vi "rethinkdb_handshake3.vi"(6 "timeout ms (10000)":i32=10000, 8 "error in (no error)":errorcluster, 10 "auth client final":string="r=rOprNGfwEbeRWgbNEkqO%hvYDpWUa2RaTCAfuxFIlj)hNlF$k0,s=W22ZaJ0SNY7soEsUEjb6gQ==,i=4096", 11 "rethinkdb in":refnum<k5>) -> (0 "error out":errorcluster, 2 "auth server final":string, 3 "rethinkdb out":refnum<k5>)   [LabVIEW 2017]
uses:
  b9d4f6d7-50ba-4a66-8241-62e1aea0d02a.vi
  17f0a6fe-6775-4334-81ae-21231bb255b8.vi
  json/rethinkdb_json_from_cluster.vi
  json/rethinkdb_json_to_cluster.vi
  json/rethinkdb_json_type_cast.vi
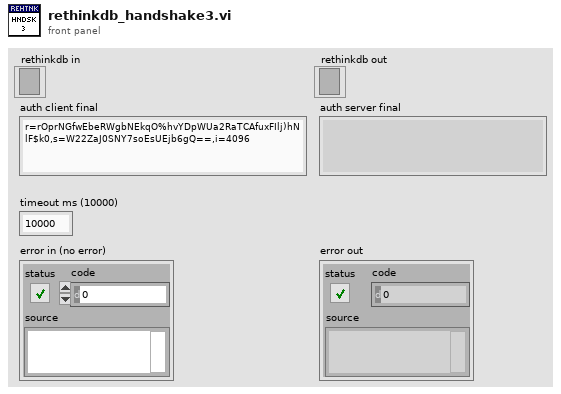
[diagram p1: front panel]
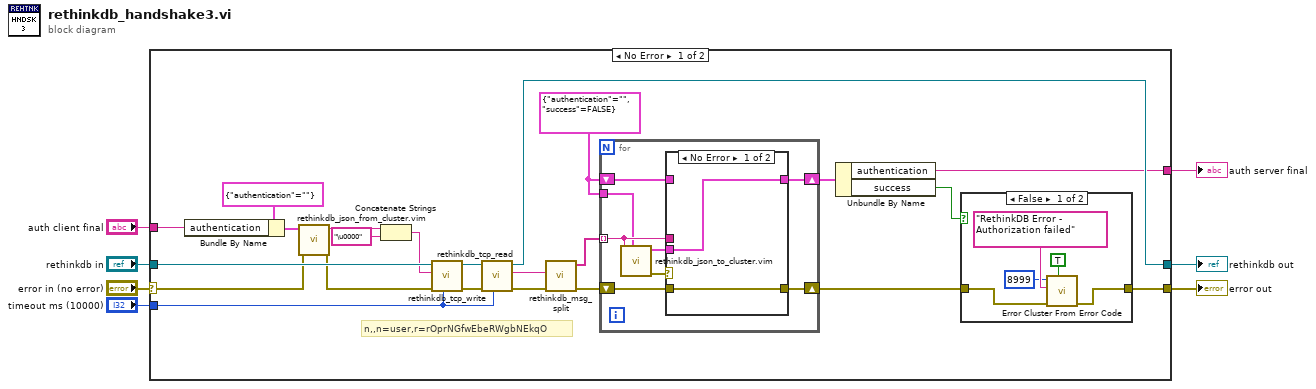
[diagram p0: block diagram]
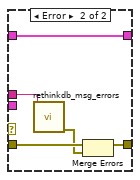
[diagram p2: hidden frame]
diagram:
  n1 = case shown="No Error" "error in (no error)" {
    selector: "error in (no error)" -> [w16 w53]
    tunnel: [w20 w53] -> w6
    tunnel: "rethinkdb in" -> [w30 w52]
    tunnel: [w23 w52] -> w4
    tunnel: "timeout ms (10000)" -> [w27 _]
    tunnel: "auth client final" -> [w11 _]
    tunnel: [w10 _] -> w1
    frame No Error {
      w17 = cluster{"authentication":string, "success":bool} {"authentication"="", "success"=FALSE} ("version")
      # "n,,n=user,r=rOprNGfwEbeRWgbNEkqO"
      n2 = Bundle By Name(cluster=cluster{"authentication":string} {"authentication"=""} ("auth_client"), "authentication"=w11) -> (w12:cluster{"authentication":string})
      n3 = call "rethinkdb_json_from_cluster.vim"("error in (no error)"=w16, "cluster"=w12) -> ("error out"=w15:errorcluster, "json"=w14:string)  [unwired: 8 in]
      n4 = Concatenate Strings(w14, "\u0000" ("string")) -> (w9:string)
      n5 = call "rethinkdb_tcp_write.vi"("timeout ms (10000)"=w27, "error in (no error)"=w15, "data in"=w9, "rethinkdb in"=w30) -> ("error out"=w29:errorcluster, "rethinkdb out"=w28:refnum<k5>)  [unwired: 5 in, 1 out]
      n6 = call "rethinkdb_tcp_read.vi"("timeout ms (10000)"=w27, "error in (no error)"=w29, "rethinkdb in"=w28) -> ("error out"=w26:errorcluster, "data out"=w22:string, "rethinkdb out"=w23:refnum<k5>)  [unwired: 6 in]
      n7 = call "rethinkdb_msg_split.vi"("error in (no error)"=w26, "data in"=w22) -> ("error out"=w25:errorcluster, "messages"=w24:string[])  [unwired: 7 in, 1 out]
      n8 = for {
        tunnel: w24 -> [w36] mode=indexing
        shift-right: [w35] -> w21
        shift-left: w17 -> [w33]
        tunnel: w17 -> [w32]
        shift-right: [w38] -> w19
        shift-left: w25 -> [w31]
        n9 = call "rethinkdb_json_to_cluster.vim"("type"=w32, "json"=w36) -> ("error out"=w37:errorcluster, "cluster"=w34:cluster{"authentication":string, "success":bool})  [unwired: 7 in, 1 out]
        n10 = case shown="No Error" w37 {
          tunnel: w36 -> [_ w44]
          tunnel: [w39 w41] -> w38
          tunnel: [w40 w45] -> w35
          tunnel: w34 -> [w40 _]
          tunnel: w33 -> [_ w45]
          tunnel: w31 -> [w39 w43]
          frame No Error {
          }
          frame Error {
            n11 = call "rethinkdb_msg_errors.vi"("message"=w44) -> ("error out"=w42:errorcluster)  [unwired: 10 in]
            n12 = Merge Errors(w43, w42) -> (w41:errorcluster)
          }
        }
      }
      n13 = Unbundle By Name(w21) -> ("authentication"=w10:string, "success"=w18:bool)
      n14 = case shown="False" w18 {
        tunnel: [w46 w51] -> w20
        tunnel: w19 -> [w47 w51]
        frame False {
          n15 = call <vilib>:"Error Cluster From Error Code.vi"("show call chain? (False)"=TRUE, "error in (no error)"=w47, "error message (\"\")"="RethinkDB Error - Authorization failed" ("error message (\"\")"), "error code (0)"=8999) -> ("error out"=w46:errorcluster)  [unwired: 5 in]
        }
        frame True {
        }
      }
    }
    frame Error {
    }
  }
  "error out" <- w6
  "rethinkdb out" <- w4
  "auth server final" <- w1
